vi "CleanUp Diagram.vi"(8 "error in (no error)":errorcluster, 10 "Top Level Diagram":refnum<vi>, 11 "Loop in":refnum<class "Loop.lvclass">) -> (0 "error out":errorcluster, 3 "Loop out":refnum<class "Loop.lvclass">)   [LabVIEW 2015, in "Loop.lvclass"]
uses:
  Loop.lvclass
  Structures/Structures.lvclass/Structures.ctl
  Loop.lvclass/Loop.ctl
  Structures/Read Structure.vi
  Read Loop Structure.vi
  Structures/Read Diagram.vi
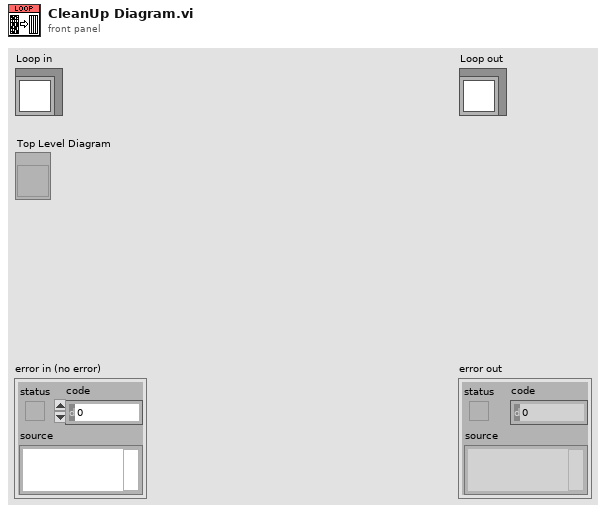
[diagram p1: front panel]
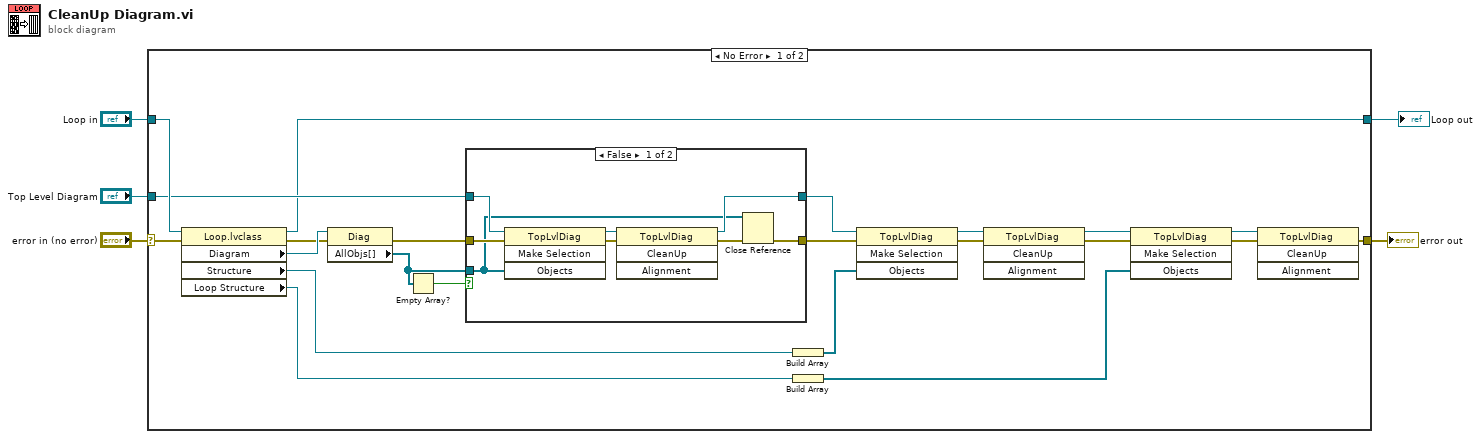
[diagram p0: block diagram]
diagram:
  n1 = case shown="No Error" "error in (no error)" {
    selector: "error in (no error)" -> [w6 w38]
    tunnel: "Loop in" -> [w10 w39]
    tunnel: "Top Level Diagram" -> [w9 _]
    tunnel: [w8 w38] -> w3
    tunnel: [w7 w39] -> w2
    frame No Error {
      n2 = property class="Loop.lvclass"(reference=w10, error in=w6) -> (reference out=w7:refnum<class "Loop.lvclass">, error out=w11:errorcluster, "Diagram"=w27:refnum<vi>, "Structure"=w12:refnum<vi>, "Loop Structure"=w14:refnum<vi>)
      n3 = property class="Diag"(reference=w27, error in=w11) -> (error out=w26:errorcluster, "AllObjs[]"=w22:refnum<vi>[])  [unwired: 1 out]
      n4 = Empty Array?(array=w22) -> (empty?=w21:bool)
      n5 = case shown="False" w21 {
        tunnel: w9 -> [w35 w36]
        tunnel: w26 -> [w32 w37]
        tunnel: [w29 w37] -> w13
        tunnel: [w31 w36] -> w24
        tunnel: w22 -> [w28 _]
        frame False {
          n6 = invoke class="TopLvlDiag" method="Make Selection"(reference=w35, error in=w32, "Objects"=w28) -> (reference out=w34:refnum<vi>, error out=w33:errorcluster)  [unwired: 1 in, 2 out]
          n7 = invoke class="TopLvlDiag" method="CleanUp"(reference=w34, error in=w33) -> (reference out=w31:refnum<vi>, error out=w30:errorcluster)  [unwired: 2 in, 2 out]
          n8 = Close Reference(reference=w28, error in (no error)=w30) -> (error out=w29:errorcluster)
        }
        frame True {
        }
      }
      n9 = Build Array(w12) -> (w20:refnum<vi>[])
      n10 = Build Array(w14) -> (w15:refnum<vi>[])
      n11 = invoke class="TopLvlDiag" method="Make Selection"(reference=w24, error in=w13, "Objects"=w20) -> (reference out=w23:refnum<vi>, error out=w25:errorcluster)  [unwired: 1 in, 2 out]
      n12 = invoke class="TopLvlDiag" method="CleanUp"(reference=w23, error in=w25) -> (reference out=w16:refnum<vi>, error out=w17:errorcluster)  [unwired: 2 in, 2 out]
      n13 = invoke class="TopLvlDiag" method="Make Selection"(reference=w16, error in=w17, "Objects"=w15) -> (reference out=w19:refnum<vi>, error out=w18:errorcluster)  [unwired: 1 in, 2 out]
      n14 = invoke class="TopLvlDiag" method="CleanUp"(reference=w19, error in=w18) -> (error out=w8:errorcluster)  [unwired: 2 in, 3 out]
    }
    frame Error {
    }
  }
  "error out" <- w3
  "Loop out" <- w2
